vi "Get Photons.vi"() -> (3 "read output":T1)   [LabVIEW 2010]
uses:
  common_typedefs/channels_cluster.ctl
  <vilib>/rvi/DataTransferAndStorage/Container/XNode/niFpgaContainer.xnode
  <vilib>/rvi/FIFO/Fifo_Resource/nirvififoEmulationSetSize.vi
  <vilib>/rvi/DataTransferAndStorage/Container/Common/niFpgaContainerGetUniqueNameForEmu.vi
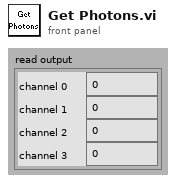
[diagram p1: front panel]
types:
  T1 = typedef "channels_cluster.ctl" = cluster{"channel 0":u32, "channel 1":u32, "channel 2":u32, "channel 3":u32}
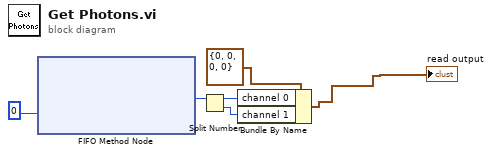
[diagram p0: block diagram]
diagram:
  n1 = xnode ("FIFO Method Node")("Timeout"=0) -> ("Element"=w4:u64)  [unwired: 1 in, 2 out]
  n2 = Split Number(x=w4) -> (hi(x)=w3:u32, lo(x)=w2:u32)
  n3 = Bundle By Name(cluster=T1 {"channel 0"=0, "channel 1"=0, "channel 2"=0, "channel 3"=0} ("read output"), "channel 0"=w3, "channel 1"=w2) -> (→"read output":T1)
